vi "HeaterStart.vi"(8 "Error In":errorcluster, 11 "VISA Resource List":string[](array[string])) -> (0 "Error Out":errorcluster, 3 "Omega CSi32 Out":refnum<visa-resource-name>)   [LabVIEW 2012]
uses:
  HeaterConfigurationGlobalAction.ctl
  libs/Omega-CSi32/Omega-CSi32.lvlib
  libs/LV-Utilities/LV-Utilities.lvlib
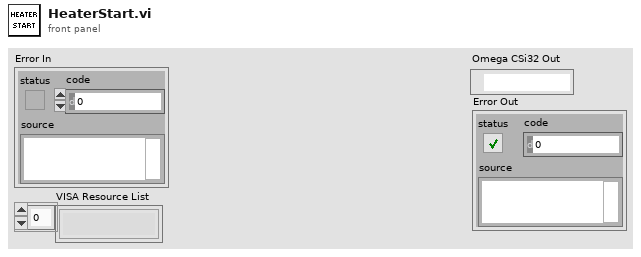
[diagram p1: front panel]
types:
  T1 = typedef "HeaterConfigurationGlobalAction.ctl" = enum16{"Init", "Get", "Set", "Add", "Remove", "Reset"}
  T2 = typedef "HeaterConfiguration.ctl" = cluster{"COM Port":u8, "Setpoint":dbl, "Standby?":bool}
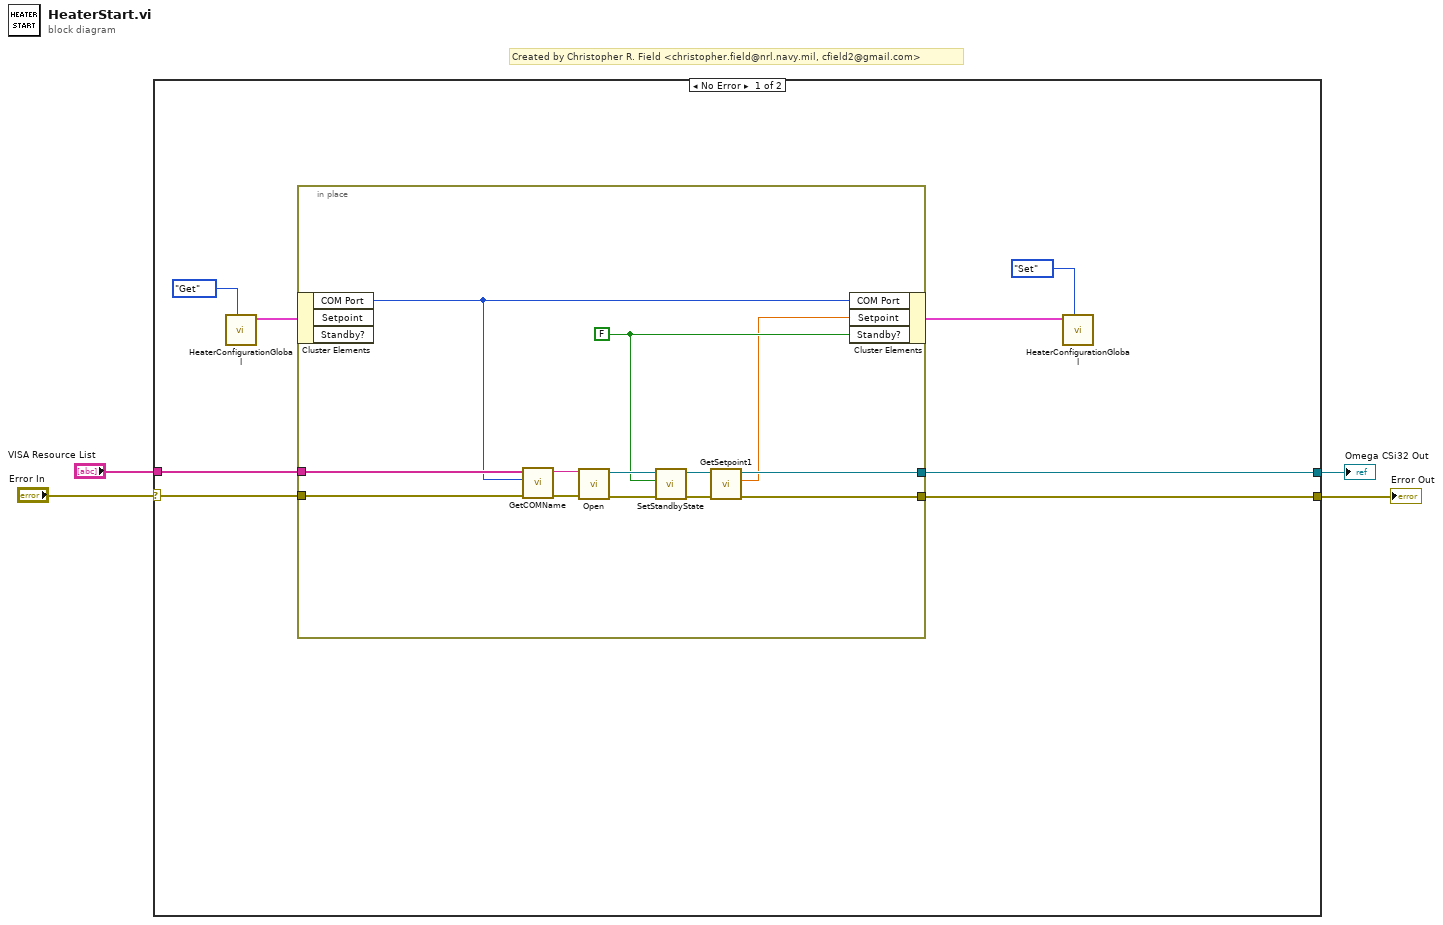
[diagram p0: block diagram]
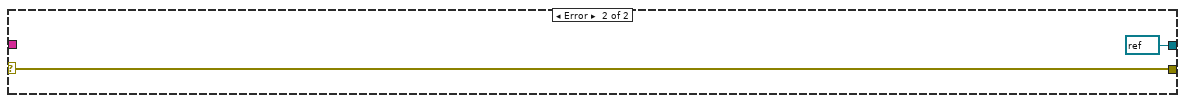
[diagram p2: hidden frame]
diagram:
  # "Created by Christopher R. Field <christopher.field@nrl.navy.mil, cfield2@gmail.com>"
  n1 = case shown="No Error" "Error In" {
    selector: "Error In" -> [w12 w27]
    tunnel: "VISA Resource List" -> [w11 _]
    tunnel: [w8 refnum<visa-resource-name> refnum ("Omega CSi32 Out")] -> w2
    tunnel: [w7 w27] -> w1
    frame No Error {
      n2 = call "HeaterConfigurationGlobal.vi"("Action"=HeaterConfigurationGlobalAction."Get") -> ("Value Out"=w6:T2)  [unwired: 10 in]
      n3 = in-place {
        in-place-border: w12 -> [w19]
        in-place-border: w11 -> [w18]
        in-place-border: [w17] -> w8
        in-place-border: [w16] -> w7
        w15 = FALSE ("Enable")
        n4 = in-place-cluster #1(w6) -> ("COM Port"=w13:u8)  [unwired: 2 out]
        n5 = call "GetCOMName.vi"("Error In"=w19, "COM Port"=w13, "VISA Resource List"=w18) -> ("Error Out"=w24:errorcluster, "VISA COM Resource Name"=w25:string)  [unwired: 6 in, 1 out]
        n6 = call "Open.vi"("Error In"=w24, "Omega CSi32 In"=w25) -> ("Error Out"=w21:errorcluster, "Omega CSi32 Out"=w20:refnum<visa-resource-name>)  [unwired: 8 in]
        n7 = call "SetStandbyState.vi"("Error In"=w21, "Enable"=w15, "Omega CSi32 In"=w20) -> ("Error Out"=w22:errorcluster, "Omega CSi32 Out"=w23:refnum<visa-resource-name>)  [unwired: 7 in]
        n8 = call "GetSetpoint1.vi"("Error In"=w22, "Omega CSi32 In"=w23) -> ("Error Out"=w16:errorcluster, "Setpoint 1 (C)"=w14:dbl, "Omega CSi32 Out"=w17:refnum<visa-resource-name>)  [unwired: 7 in]
        n9 = in-place-cluster #1("COM Port"=w13, "Setpoint"=w14, "Standby?"=w15) -> (w5:T2)
      }
      n10 = call "HeaterConfigurationGlobal.vi"("Action"=HeaterConfigurationGlobalAction."Set", "Set Value"=w5) -> ()  [unwired: 9 in, 1 out]
    }
    frame Error {
    }
  }
  "Omega CSi32 Out" <- w2
  "Error Out" <- w1
